vi "Flatness_Load-CalFromStep.vi"(8 "error in":errorcluster {"code" format="%.0x"}, 11 "Session In":refnum<visa-resource-name>="TCPIP0::169.254.70.100::inst0::INSTR") -> (0 "error out":errorcluster {"code" format="%.0x"}, 3 "Session Out":refnum<visa-resource-name>)   [LabVIEW 2018]
doc: "Launches the Instrument I/O Assistant, which you can use to communicate with message-based instruments and graphically parse the response. For example you can communicate with an instrument that uses a serial, Ethernet, or GPIB interface."
panel:
  in  "Timeout":u32=3000
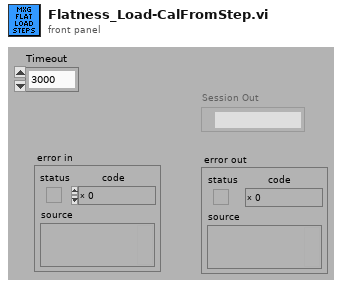
[diagram p1: front panel]
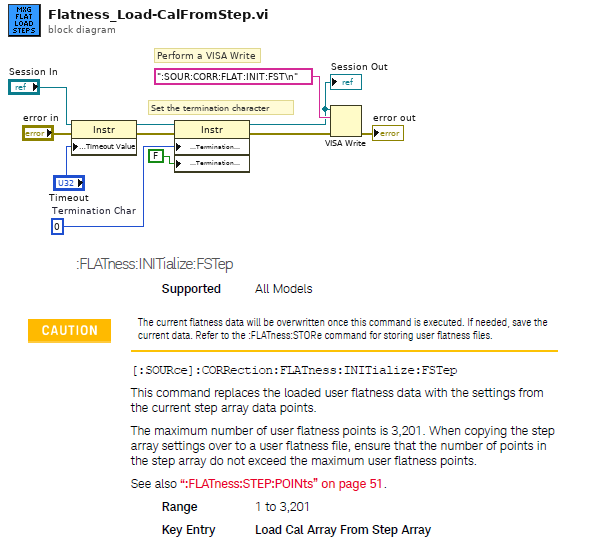
[diagram p0: block diagram]
diagram:
  w6 = u8 0  # Termination Char
  # "Perform a VISA Write"
  # "Set the termination character"
  n1 = property class="Instr"(reference="Session In", error in="error in", "General Settings:Timeout Value"="Timeout") -> (reference out=w5:refnum<visa-resource-name>, error out=w8:errorcluster)
  n2 = property class="Instr"(reference=w5, error in=w8, "Message Based Settings:Termination Character"=w6, "Message Based Settings:Termination Character Enable"=FALSE ("enable")) -> (reference out=w1:refnum<visa-resource-name>, error out=w7:errorcluster)
  "Session Out" <- w1
  n3 = VISA Write(VISA resource name=w1, write buffer=":SOUR:CORR:FLAT:INIT:FST\n" ("StaticText"), error in (no error)=w7) -> (error out=→"error out":errorcluster)  [unwired: 2 out]
